vi "Initialize.vi"(8 "error in (no error)":errorcluster, 10 "Reply to":refnum<class "Result Reply Msg.lvclass">, 11 "Measure Object in":refnum<class "Measure Object.lvclass">) -> (0 "error out":errorcluster, 3 "Measure Object out":refnum<class "Measure Object.lvclass">)   [LabVIEW 2015, in "Measure Object.lvclass"]
uses:
  Measure Object.lvclass
  Measure Object Messages/Result Reply Msg/Result Reply Msg.lvclass
  Measure Object.lvclass/Measure Object.ctl
  Results/Acquired Result/Acquired Result.lvclass/Acquired Result.ctl
  Results/Acquired Result/Write Sender.vi
  Results/Acquired Result/Acquired Result.lvclass
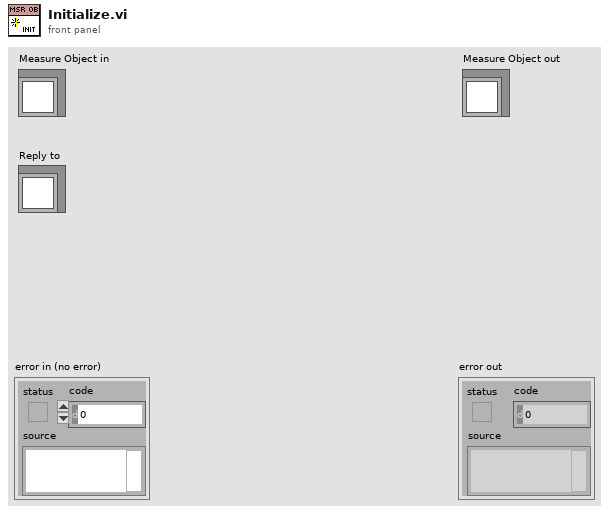
[diagram p1: front panel]
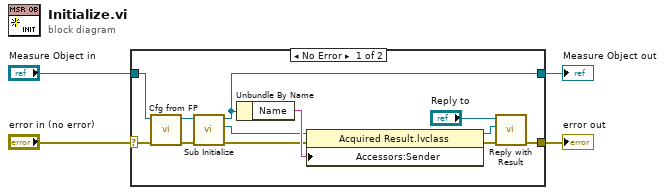
[diagram p0: block diagram]
diagram:
  n1 = case shown="No Error" "error in (no error)" {
    selector: "error in (no error)" -> [w9 w18]
    tunnel: [w16 w18] -> w3
    tunnel: [w8 w17] -> w1
    tunnel: "Measure Object in" -> [w15 w17]
    frame No Error {
      n2 = call-dynamic "Cfg from FP.vi"("error in (no error)"=w9, "Measure Object in"=w15) -> ("error out"=w6:errorcluster, "Measure Object out"=w10:refnum<class "Measure Object.lvclass">)  [unwired: 8 in]
      n3 = call-dynamic "Sub Initialize.vi"("error in (no error)"=w6, "Measure Object in"=w10) -> ("error out"=w5:errorcluster, "Initialize Result"=w7:refnum<class "Acquired Result.lvclass">, "Measure Object out"=w8:refnum<class "Measure Object.lvclass">)  [unwired: 7 in]
      n4 = Unbundle By Name(w8) -> ("Name"=w14:string)
      n5 = property class="Acquired Result.lvclass"(reference=w7, error in=w5, "Accessors:Sender"=w14) -> (reference out=w11:refnum<class "Acquired Result.lvclass">, error out=w13:errorcluster)
      n6 = call-dynamic "Reply with Result.vi"("error in (no error)"=w13, "Result"=w11, "Result Reply Msg in"="Reply to") -> ("error out"=w16:errorcluster)  [unwired: 7 in, 1 out]
    }
    frame Error {
    }
  }
  "error out" <- w3
  "Measure Object out" <- w1
